vi "MODBUS_CRC16.vi"(11 "String":string) -> (2 "CRC-16 2":string, 3 "String & CRC-16":string)   [LabVIEW 2014]
panel:
  out "CRC-16":u8
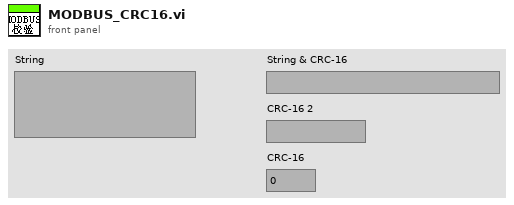
[diagram p1: front panel]
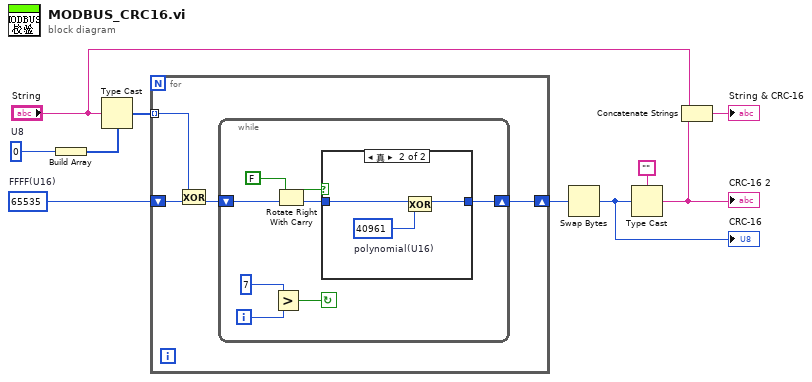
[diagram p0: block diagram]
diagram:
  w2 = u16 65535  # FFFF(U16)
  w10 = u8 0  # U8
  n1 = Build Array(w10) -> (w9:u8[])
  n2 = Type Cast(type=w9, x="String") -> (*(type *) &x=w8:u8[])
  n3 = for {
    tunnel: w8 -> [w14] mode=indexing
    shift-right: [w11] -> w1
    shift-left: w2 -> [w13]
    n4 = Exclusive Or(1:w13, 2:w14) -> (0:w12:u16)
    n5 = while {
      shift-right: [w18] -> w11
      shift-left: w12 -> [w16]
      i -> [w17]
      stop <- w15 continue-if-true
      n6 = Greater?(x=7, y=w17) -> (0:w15:bool)
      n7 = Rotate Right With Carry(2:w16, 3:FALSE) -> (0:w19:u16, 1:w20:bool)
      n8 = case shown="真" w20 {
        tunnel: w19 -> [w23 w26]
        tunnel: [w23 w24] -> w18
        frame False {
        }
        frame True {
          w25 = u16 40961  # polynomial(U16)
          n9 = Exclusive Or(1:w25, 2:w26) -> (0:w24:u16)
        }
      }
    }
  }
  n10 = Swap Bytes(anything=w1) -> (byte swapped=w7:u16)
  "CRC-16" <- w7
  n11 = Type Cast(type="", x=w7) -> (*(type *) &x=w5:string)
  "CRC-16 2" <- w5
  n12 = Concatenate Strings("String", w5) -> (→"String & CRC-16":string)
